vi "DSF.Engine.Buffer Converter.Initialize Data Type Buffers.vi"(8 "error in (no error)":errorcluster, 10 "channel count (1M)":i32=1000000, 11 "Buffer Converter in":refnum<class "Buffer Converter.lvclass">) -> (0 "error out":errorcluster, 3 "Buffer Converter out":refnum<class "Buffer Converter.lvclass">)   [LabVIEW 2017, in "DSF.Engine.lvlib" / "Buffer Converter.lvclass"]
uses:
  Buffer Converter.lvclass
  Shared/Typedefs/DSF.Shared.Typedefs.Type Buffers.ctl
  Buffer Converter.lvclass/Buffer Converter.ctl
  DSF.Engine.lvlib
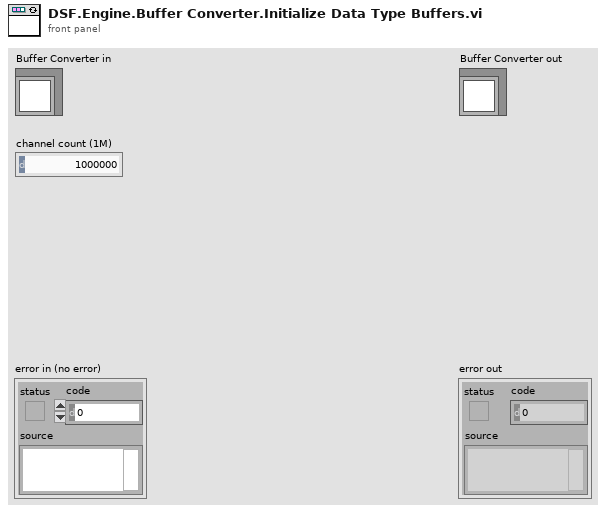
[diagram p1: front panel]
types:
  T1 = typedef "DSF.Engine.lvlib/DSF.Shared.Typedefs.Type Buffers.ctl" = cluster{"Bool":bool[], "SGL":sgl[], "DBL":dbl[], "I8":i8[], "I16":i16[], "I32":i32[], "I64":i64[], "U8":u8[], "U16":u16[], "U32":u32[], "U64":u64[]}
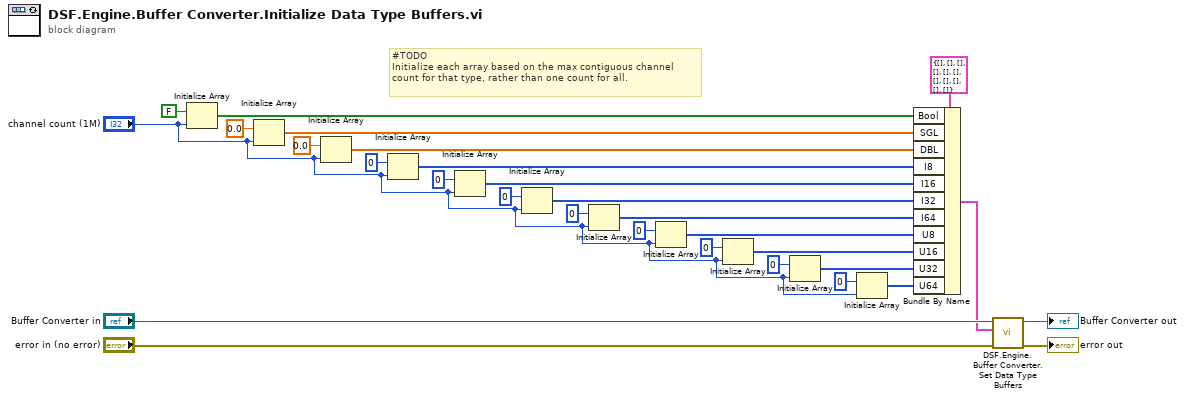
[diagram p0: block diagram]
diagram:
  # "#TODO\nInitialize each array based on the max contiguous channel count for that type, rather than one count for all."
  n1 = Initialize Array(FALSE, "channel count (1M)") -> (w25:bool[])
  n2 = Initialize Array(sgl 0.0, "channel count (1M)") -> (w24:sgl[])
  n3 = Initialize Array(0.0, "channel count (1M)") -> (w21:dbl[])
  n4 = Initialize Array(i8 0, "channel count (1M)") -> (w6:i8[])
  n5 = Initialize Array(i16 0, "channel count (1M)") -> (w7:i16[])
  n6 = Initialize Array(0, "channel count (1M)") -> (w8:i32[])
  n7 = Initialize Array(i64 0, "channel count (1M)") -> (w9:i64[])
  n8 = Initialize Array(u8 0, "channel count (1M)") -> (w10:u8[])
  n9 = Initialize Array(u16 0, "channel count (1M)") -> (w11:u16[])
  n10 = Initialize Array(u32 0, "channel count (1M)") -> (w12:u32[])
  n11 = Initialize Array(u64 0, "channel count (1M)") -> (w13:u64[])
  n12 = Bundle By Name(cluster=T1 {"Bool"=[], "SGL"=[], "DBL"=[], "I8"=[], "I16"=[], "I32"=[], "I64"=[], "U8"=[], "U16"=[], "U32"=[], "U64"=[]} ("Data Type Buffers"), "Bool"=w25, "SGL"=w24, "DBL"=w21, "I8"=w6, "I16"=w7, "I32"=w8, "I64"=w9, "U8"=w10, "U16"=w11, "U32"=w12, "U64"=w13) -> (w3:T1)
  n13 = call "DSF.Engine.Buffer Converter.Set Data Type Buffers.vi"("data type buffers"=w3, "Buffer Converter in"="Buffer Converter in") -> ("Buffer Converter out"=→"Buffer Converter out":refnum<class "Buffer Converter.lvclass">)  [unwired: 9 in]
  "error out" <- "error in (no error)"
